vi "Log Results.vi"(8 "error in (no error)":errorcluster, 11 "Instrument.Lockin in":refnum<class "Instrument.Lockin.lvclass">) -> (0 "error out":errorcluster, 3 "Instrument.Lockin out":refnum<class "Instrument.Lockin.lvclass">)   [LabVIEW 2019, in "Instrument.Lockin.lvlib" / "Instrument.Lockin.lvclass"]
uses:
  Instrument.Lockin.lvclass
  C:/Program Files/National Instruments/LabVIEW 2019/user.lib/LevyLab/Instrument Framework/Instrument/Instrument.lvclass
  Instrument.Lockin.lvclass/Instrument.Lockin.ctl
  Typedefs/Results Type--Enum.ctl
  <userlib>/LevyLab/Instrument Framework/Instrument/Instrument.lvclass
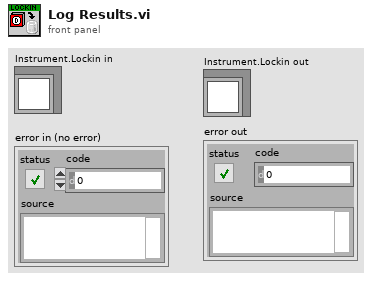
[diagram p1: front panel]
types:
  T1 = typedef "Instrument.Lockin.lvlib/Instrument.Lockin.lvclass/Results Type--Enum.ctl" = enum16{"X", "Y", "R", "Theta", "Mean"}
  T2 = typedef "Instrument.Lockin.lvlib/Instrument.DAQ.lvclass/DeviceInfo--Cluster.ctl" = cluster{"DeviceName":string, "DevIsSimulated":bool, "DeviceSerialNumber":u32, "ProductType":string, "ProductCategory":i32, "ProductNumber":u32, "ChassisNumber":u32, "SlotNumber":u32, "ChassisName":string, "ChassisSerialNumber":u32}
  T3 = typedef "Instrument.Lockin.lvlib/Instrument.DAQ.lvclass/Results--Cluster.ctl" = cluster{"Time Stamp":timestamp, "Results (Dictionary)":cluster{"key":string, "value":dbl}[]}
  T4 = cluster{"ChassisSerialNumber":u32, i32, i32, dbl, dbl, bool}
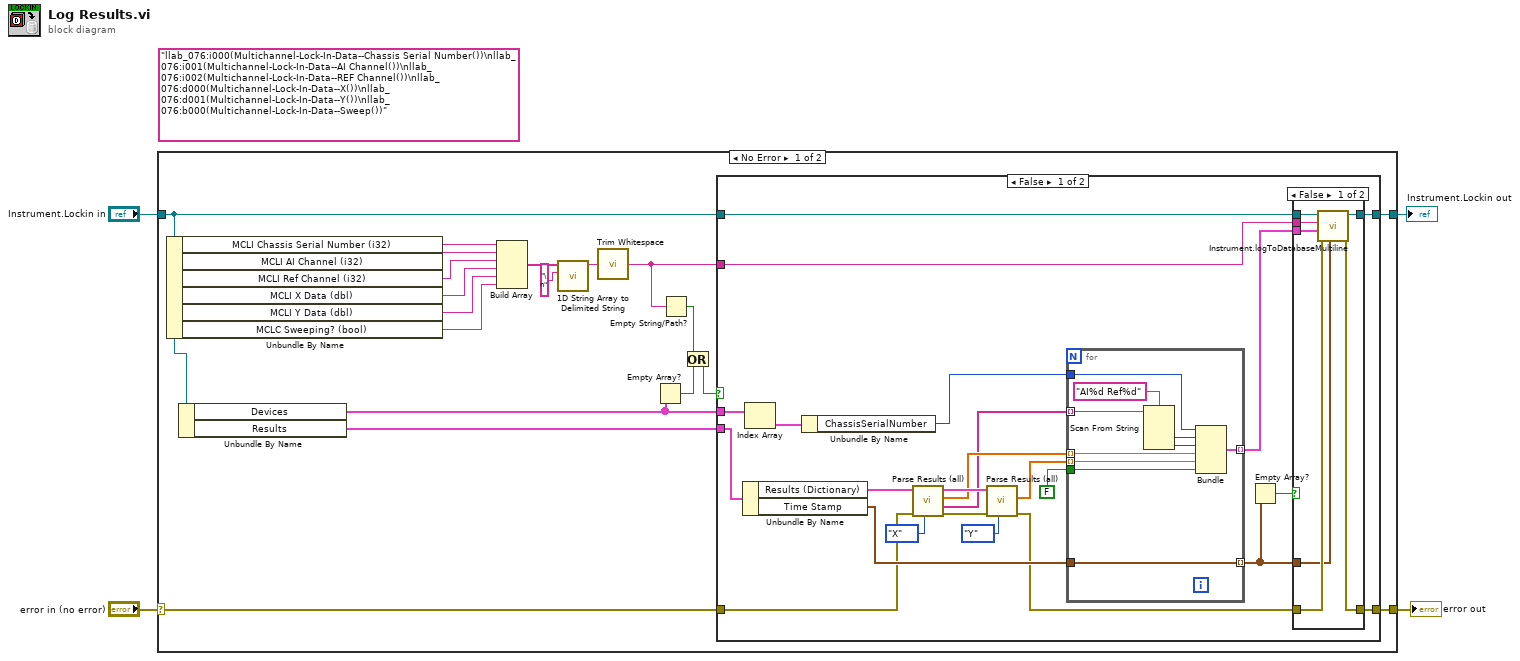
[diagram p0: block diagram]
diagram:
  (unwired) "llab_076:i000(Multichannel-Lock-In-Data--Chassis Serial Number())\nllab_076:i001(Multichannel-Lock-In-Data--AI Channel())\nllab_076:i002(Multichannel-Lock-In-Data--REF Channel())\nllab_076:d000(Multichannel-Lock-In-Data--X())\nllab_076:d001(Multichannel-Lock-In-Data--Y())\nllab_076:b000(Multichannel-Lock-In-Data--Sweep())"
  n1 = case shown="No Error" "error in (no error)" {
    selector: "error in (no error)" -> [w22 w69]
    tunnel: "Instrument.Lockin in" -> [w19 w68]
    tunnel: [w23 w69] -> w3
    tunnel: [w7 w68] -> w1
    frame No Error {
      n2 = Unbundle By Name(w19) -> ("MCLI Chassis Serial Number (i32)"=w13:string, "MCLI AI Channel (i32)"=w18:string, "MCLI Ref Channel (i32)"=w17:string, "MCLI X Data (dbl)"=w16:string, "MCLI Y Data (dbl)"=w15:string, "MCLC Sweeping? (bool)"=w14:string)
      n3 = Unbundle By Name(w19) -> ("Devices"=w20:T2[], "Results"=w21:T3)
      n4 = Build Array(w13, w18, w17, w16, w15, w14) -> (w12:string[])
      n5 = call <vilib>:"1D String Array to Delimited String.vi"("delimiter"="\n", "string array"=w12) -> ("delimited string"=w6:string)  [unwired: 9 in]
      n6 = call <vilib>:"Trim Whitespace.vi"("string"=w6) -> ("trimmed string"=w5:string)  [unwired: 1 in]
      n7 = Empty Array?(array=w20) -> (empty?=w10:bool)
      n8 = Empty String/Path?(string/path=w5) -> (empty?=w8:bool)
      n9 = Or(x=w8, y=w10) -> (x .or. y?=w9:bool)
      n10 = case shown="False" w9 {
        tunnel: w19 -> [w46 w66]
        tunnel: [w45 w67] -> w23
        tunnel: w22 -> [w28 w67]
        tunnel: w21 -> [w31 _]
        tunnel: w20 -> [w32 _]
        tunnel: w5 -> [w25 _]
        tunnel: [w24 w66] -> w7
        frame False {
          n11 = Unbundle By Name(w31) -> ("Results (Dictionary)"=w44:cluster{"key":string, "value":dbl}[], "Time Stamp"=w30:timestamp)
          n12 = Index Array(array=w32) -> (element=w34:T2)  [unwired: 1 in]
          n13 = Unbundle By Name(w34) -> ("ChassisSerialNumber"=w36:u32)
          n14 = call "Parse Results (all).vi"("Type"=Results_Type--Enum."X", "error in (no error)"=w28, "Results (Dictionary)"=w44) -> ("error out"=w40:errorcluster, "Names"=w37:string[], "Data"=w38:dbl[], "Results (Dictionary)"=w41:cluster{"key":string, "value":dbl}[])  [unwired: 5 in]
          n15 = call "Parse Results (all).vi"("Type"=Results_Type--Enum."Y", "error in (no error)"=w40, "Results (Dictionary)"=w41) -> ("error out"=w29:errorcluster, "Data"=w39:dbl[])  [unwired: 5 in, 2 out]
          n16 = for {
            tunnel: w36 -> [w56]
            tunnel: w38 -> [w55] mode=indexing
            tunnel: w39 -> [w54] mode=indexing
            tunnel: w37 -> [w50] mode=indexing
            tunnel: [w49] -> w27 mode=indexing
            tunnel: w30 -> [w48]
            tunnel: [w48] -> w33 mode=indexing
            tunnel: FALSE -> [w47]
            n17 = Scan From String(format string="AI%d Ref%d", input string=w50) -> (output 1=w52:i32, output 2=w51:i32)  [unwired: 4 in, 3 out]
            n18 = Bundle("ChassisSerialNumber"=w56, w52, w51, w55, w54, w47) -> (w49:T4)  [unwired: 1 in]
          }
          n19 = Empty Array?(array=w33) -> (empty?=w26:bool)
          n20 = case shown="False" w26 {
            tunnel: w46 -> [w63 w64]
            tunnel: [w62 w65] -> w45
            tunnel: w29 -> [w61 w65]
            tunnel: w25 -> [w60 _]
            tunnel: w27 -> [w59 _]
            tunnel: w33 -> [w58 _]
            tunnel: [w57 w64] -> w24
            frame False {
              n21 = call <userlib>:"Instrument.logToDatabaseMultiline.vi"("timestamps"=w58, "error in (no error)"=w61, "Data"=w59, "Paths"=w60, "Instrument"=w63) -> ("error out"=w62:errorcluster, "Instrument out"=w57:refnum<class "Instrument.Lockin.lvclass">)  [unwired: 5 in]
            }
            frame True {
            }
          }
        }
        frame True {
        }
      }
    }
    frame Error {
    }
  }
  "error out" <- w3
  "Instrument.Lockin out" <- w1
